vi "Main_camera_2.vi"() -> ()   [LabVIEW 2023]
uses:
  <vilib>/userDefined/High Color/IMAQdx.ctl
  <vilib>/vision/driver/NI_Vision_Acquisition_Software.lvlib
  <resource>/objmgr/imaqdx.rc
panel:
  in  "Starting acquisition \ndelay in seconds":dbl
  in  "seconds\n between acquistions":u32
  in  "Object Parameters Attributes":T1={"ReflectedTemperature"=300.0, "AtmosphericTemperature"=300.0, "ExtOpticsTemperature"=300.0, "ObjectEmissivity "=0.95, "RelativeHumidity "=1.0, "ExtOpticsTransmission"=1.0, "EstimatedTransmission"=0.0, "ObjectDistance"=0.0} {"ObjectDistance" min=0.0 max=10000.0 step=1.0; "EstimatedTransmission" min=0.0 max=1.0 step=0.01; "ExtOpticsTransmission" min=0.0 max=1.0 step=0.01; "RelativeHumidity" min=0.0 max=1.0 step=0.01; "ObjectEmissivity" min=0.0 max=1.0 step=0.01; "ExtOpticsTemperature" min=0.0 max=5000.0 step=1.0; "AtmosphericTemperature" min=0.0 max=5000.0 step=1.0; "ReflectedTemperature" min=0.0 max=5000.0 step=1.0}
  in  "PacketSize":u32=1500
  in  "NUCMode":enum16{"Off", "On"}(ring)=enum."On"
  in  "IRFormat":i64(ring)=1 items=["Radiometric", "TemperatureLinear100mK", "TemperatureLinear10mK"]
  out "Image":T2(plugin-control)
  in  "Stop":bool
  # "Please select the camera you want to access the thermal image\ncamera connected to ethernet port 1 -> cam0"
  # "Note: The Image control needs to be set to 16-bit display. This is done by with the following steps\n            1) Right click on the Image display and select 16-Bit Display Mapping to bring up Set 16 Bit Display Mapping window\n            2) Un-tick \"Apply mapping only when Configured bit depth is 0\" in the Set 16 Bit Display Mapping window\n            3) Set the Conversion Method to Full Dynamic if not already selected"
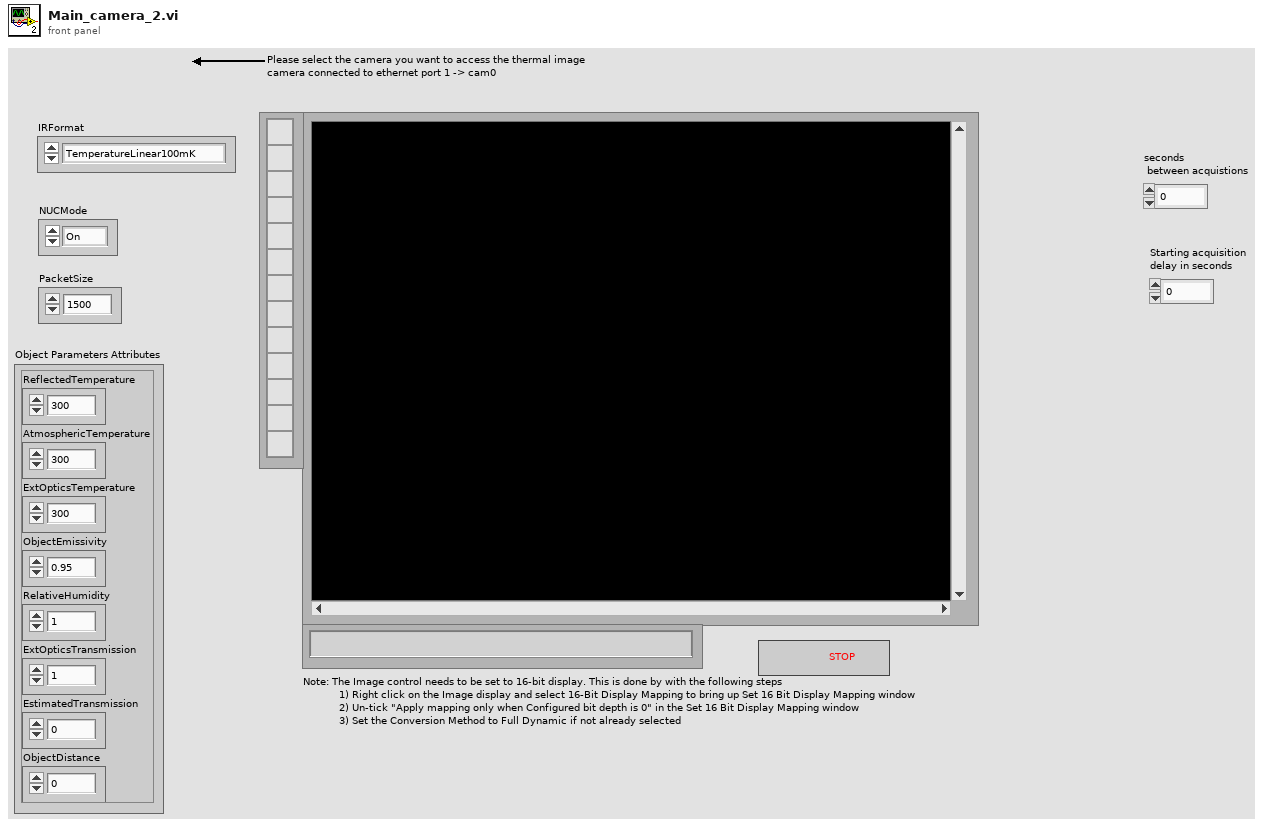
[diagram p1: front panel]
types:
  T1 = cluster{"ReflectedTemperature":dbl, "AtmosphericTemperature":dbl, "ExtOpticsTemperature":dbl, "ObjectEmissivity ":dbl, "RelativeHumidity ":dbl, "ExtOpticsTransmission":dbl, "EstimatedTransmission":dbl, "ObjectDistance":dbl}
  T2 = typedef "IMAQ Image.ctl" = refnum<image>
  T3 = typedef "IMAQdx.ctl" = refnum<k21>
  T4 = typedef "Image Type" = u32
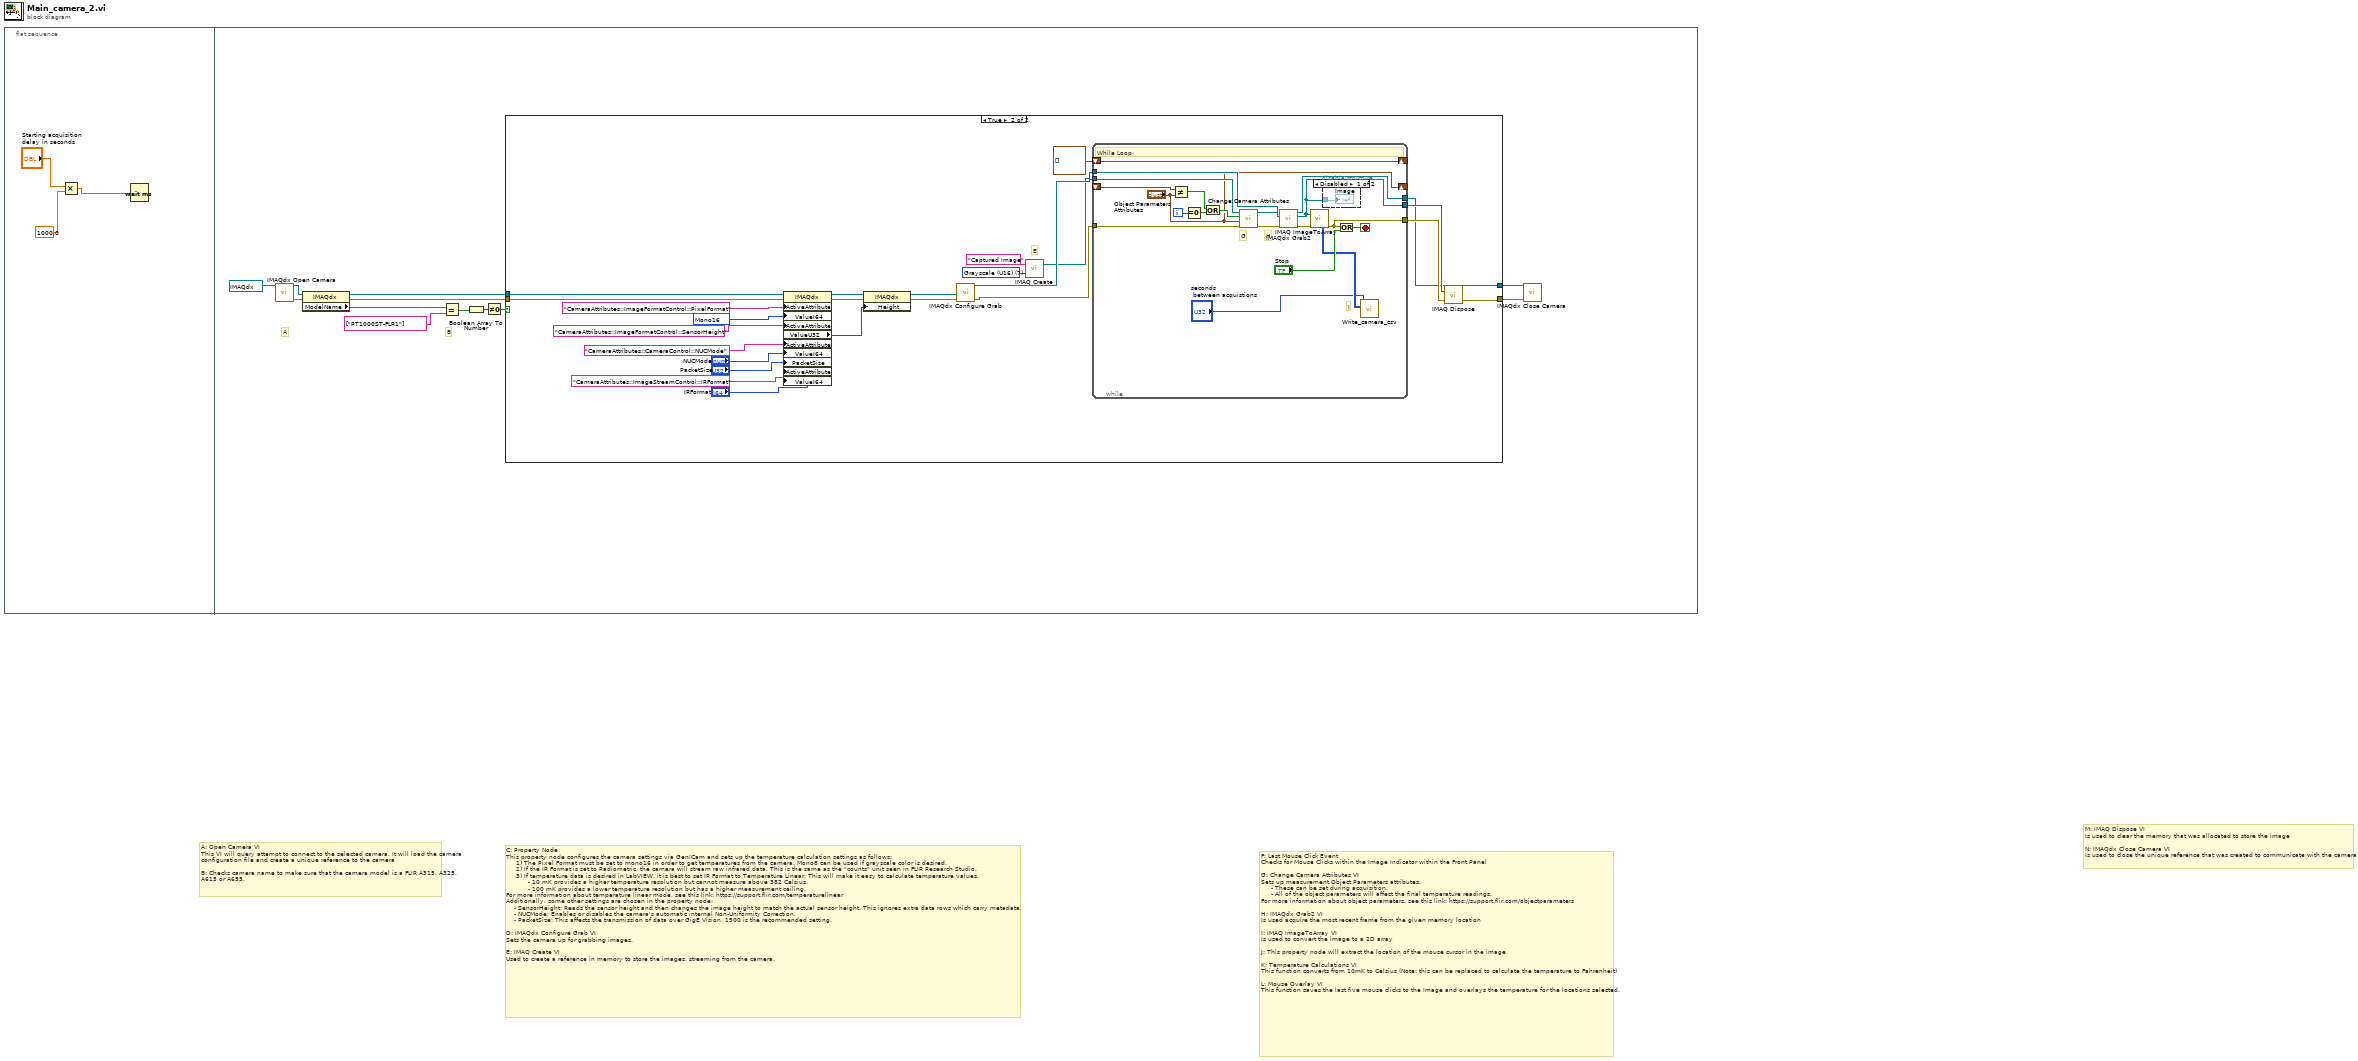
[diagram p0: block diagram]
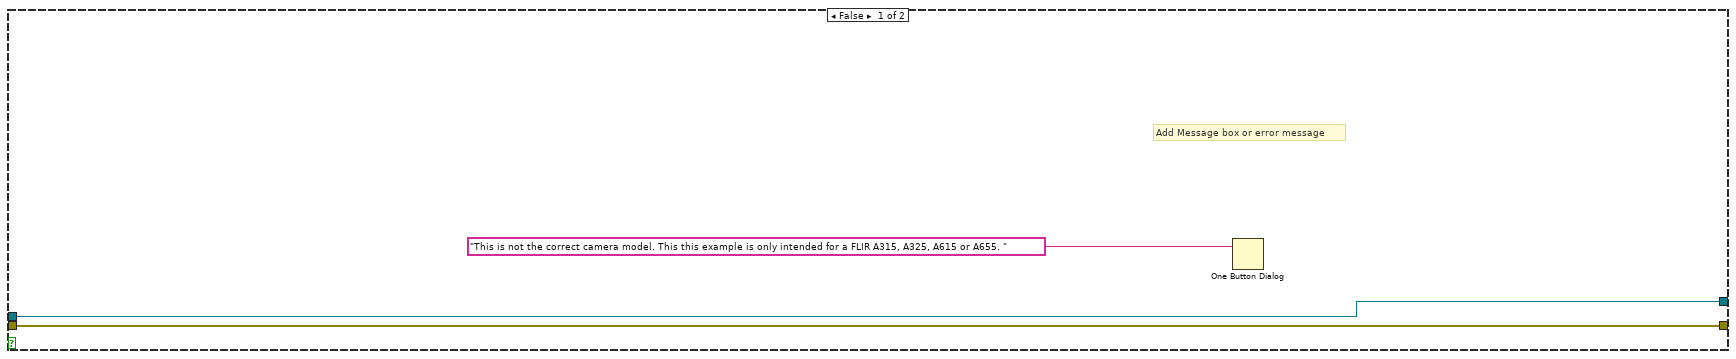
[diagram p2: hidden frame]
diagram:
  # "M: IMAQ Dispose VI\nIs used to clear the memory that was allocated to store the image\n\nN: IMAQdx Close Camera VI\nIs used to close the unique reference that was created to communicate with the camera"
  # "F: Last Mouse Click Event\nChecks for Mouse Clicks within the Image Indicator within the Front Panel \n\nG: Change Camera Attributes VI \nSets up measurement Object Parameters attributes. \n     - These can be set during acquisition. \n     - All of the object parameters will affect the final temperature readings. \nFor more information about object parameters, see this link: https://support.flir.com/objectparameters\n\nH: IMAQdx Grab2 VI\nIs used acquire the most recent frame from the given memory location\n\nI: IMAQ ImageToArray VI\nIs used to convert the image to a 2D array\n\nJ: This property node will extract the location of the mouse cursor in the image\n\nK: Temperature Calculations VI \nThis function converts from 10mK to Celsius (Note: this can be replaced to calculate the temperature to Fahrenheit)\n\nL: Mouse Overlay VI\nThis function saves the last five mouse clicks to the Image and overlays the temperature for the locations selected."
  # "A: Open Camera VI\nThis VI will query attempt to connect to the selected camera. It will load the camera configuration file and create a unique reference to the camera\n\nB: Checks camera name to make sure that the camera model is a FLIR A315, A325, A615 or A655."
  # "C: Property Node\nThis property node configures the camera settings via GenICam and sets up the temperature calculation settings as follows: \n     1) The Pixel Format must be set to mono16 in order to get temperatures from the camera. Mono8 can be used if grayscale color is desired.\n     2) If the IR Format is set to Radiometric, the camera will stream raw infrared data. This is the same as the \"counts\" unit seen in FLIR Research Studio.\n     3) If temperature data is desired in LabVIEW, it is best to set IR Format to Temperature Linear. This will make it easy to calculate temperature values.\n           - 10 mK provides a higher temperature resolution but cannot measure above 382 Celsius.\n           - 100 mK provides a lower temperature resolution but has a higher measurement ceiling.\nFor more information about temperature linear mode, see this link: https://support.flir.com/temperaturelinear\nAdditionally, some other settings are chosen in the property node:\n    - SensorHeight: Reads the sensor height and then changes the image height to match the actual sensor height. This ignores extra data rows which carry metadata.\n    - NUCMode: Enables or disables the camera's automatic internal Non-Uniformity Correction. \n    - PacketSize: This affects the transmission of data over GigE Vision. 1500 is the recommended setting. \n\nD: IMAQdx Configure Grab VI\nSets the camera up for grabbing images.\n\nE: IMAQ Create VI\nUsed to create a reference in memory to store the images, streaming from the camera."
  n1 = flat-sequence {
    frame #0 {
      n2 = Multiply(x="Starting acquisition \ndelay in seconds", y=1000.0) -> (x*y=w1:dbl)
      n3 = Wait (ms)(milliseconds to wait=w1) -> ()  [unwired: 1 out]
    }
    frame #1 {
      # "B"
      # "A"
      n4 = call <vilib>:"IMAQdx Open Camera.vi"("Session In"=T3 "cam0") -> ("error out"=w12:errorcluster, "Session Out"=w13:T3)  [unwired: 9 in]
      n5 = property class="IMAQdx"(reference=w13, error in=w12) -> (reference out=w11:T3, error out=w10:errorcluster, "ModelName"=w9:string)
      n6 = Equal?(x=w9, y=string[] ["PT1000ST-FLR1"]) -> (x = y?=w6:bool[])
      n7 = Boolean Array To Number(Boolean array=w6) -> (number=w7:u32)
      n8 = Not Equal To 0?(x=w7) -> (x != 0?=w5:bool)
      n9 = case shown="True" w5 {
        tunnel: [w17 w39] -> w15
        tunnel: [w18 w36] -> w14
        tunnel: w11 -> [w18 w35]
        tunnel: w10 -> [w17 w34]
        frame False {
          # "Add Message box or error message"
          n10 = One Button Dialog(message="This is not the correct camera model. This this example is only intended for a FLIR A315, A325, A615 or A655. ") -> ()  [unwired: 1 in, 1 out]
        }
        frame True {
          w32 = i64 17825799 items=["Mono 8"=17301505, "Mono8Signed"=17301506, "Mono10"=17825795, "Mono10Packed"=17563652, "Mono12"=17825797, "Mono12Packed"=17563654, "Mono16"=17825799] ("Ring")
          w42 = T4 7 items=["Grayscale (U8)", "Grayscale (I16)", "Grayscale (SGL)", "Complex (CSG)", "RGB (U32)", "HSL (U32)", "RGB (U64)", "Grayscale (U16)"] ("Image Type")
          # "E"
          n11 = property class="IMAQdx"(reference=w35, error in=w34, "ActiveAttribute"="CameraAttributes::ImageFormatControl::PixelFormat", "ValueI64"=w32, "ActiveAttribute"="CameraAttributes::ImageFormatControl::SensorHeight", "ActiveAttribute"="CameraAttributes::CameraControl::NUCMode", "ValueI64"="NUCMode", "PacketSize"="PacketSize", "ActiveAttribute"="CameraAttributes::ImageStreamControl::IRFormat", "ValueI64"="IRFormat") -> (reference out=w24:T3, error out=w22:errorcluster, "ValueU32"=w19:u32)
          n12 = property class="IMAQdx"(reference=w24, error in=w22, "Height"=w19) -> (reference out=w23:T3, error out=w21:errorcluster)
          n13 = call <vilib>:"IMAQdx Configure Grab.vi"("error in"=w21, "Session In"=w23) -> ("error out"=w26:errorcluster, "Session Out"=w41:T3)  [unwired: 8 in]
          n14 = call "IMAQ Create"("Image Name"="Captured Image", "Image Type"=w42) -> ("New Image"=w40:T2)  [unwired: 3 in, 1 out]
          n15 = while {
            tunnel: [w47] -> w37
            tunnel: [w46] -> w38
            shift-right: [w48] -> _
            shift-left: cluster{"X":i32, "Y":i32}[] [] ("Array In") -> [w48]
            tunnel: w41 -> [w59]
            tunnel: w26 -> [w44]
            tunnel: w40 -> [w61]
            tunnel: [w60] -> w36
            shift-right: ["Object Parameters Attributes"] -> _
            shift-left: _ -> [w51]
            i -> [w56]
            stop <- w63 stop-if-true
            # "I"
            # "H"
            # "G"
            # "While Loop"
            n16 = Not Equal?(x=w51, y="Object Parameters Attributes") -> (x != y?=w54:bool)
            n17 = Equal To 0?(x=w56) -> (x = 0?=w55:bool)
            n18 = Or(x=w54, y=w55) -> (x .or. y?=w53:bool)
            n19 = call "Change Camera Attributes.vi"("error in"=w44, "Object Parameters Attributes"="Object Parameters Attributes", "Boolean"=w53, "Session In"=w59) -> ("error out"=w58:errorcluster, "Session Out"=w57:T3)  [unwired: 6 in]
            n20 = call <vilib>:"IMAQdx Grab2.vi"("error in"=w58, "Image In"=w61, "Session In"=w57) -> ("error out"=w52:errorcluster, "Image Out"=w46:T2, "Session Out"=w60:T3)  [unwired: 5 in, 1 out]
            n21 = call "IMAQ ImageToArray"("error in (no error)"=w52, "Image"=w46) -> ("Image Pixels (U16)"=w49:u16[][], "error out"=w47:errorcluster)  [unwired: 2 in, 3 out]
            n22 = disable-structure shown="Disabled" {
              disable-tunnel: w46 -> [w64 _]
              frame Disabled {
                "Image" <- w64
              }
              frame Enabled {
              }
            }
            n23 = Or(x=w47, y="Stop") -> (x .or. y?=w63:bool)
            n24 = call "Write_camera_csv.vi"("Image Pixels (U16)"=w49, "seconds\n between acquistions"="seconds\n between acquistions") -> ()  [unwired: 10 in]
          }
          n25 = call "IMAQ Dispose"("Image"=w38, "error in (no error)"=w37) -> ("error out"=w39:errorcluster)  [unwired: 4 in]
        }
      }
      n26 = call <vilib>:"IMAQdx Close Camera.vi"("error in"=w15, "Session In"=w14) -> ()  [unwired: 9 in, 1 out]
    }
  }
